vi "FINAL PROJECT PRO .vi"() -> ()   [LabVIEW 2015]
uses:
  <vilib>/LabVIEW Interface for Arduino/Type Defs/Board Type.ctl
  <vilib>/LabVIEW Interface for Arduino/Type Defs/Connection Type.ctl
  <vilib>/LabVIEW Interface for Arduino/Type Defs/Pin Mode.ctl
  <vilib>/Instr/_visa.llb/VISA Configure Serial Port (Instr).vi
  <vilib>/LabVIEW Interface for Arduino/LabVIEW Interface for Arduino.lvlib
panel:
  out "DISPLAY MESSAGE":string
  out "TRANSACTION PROCESSING":string
  out "ARDUINO GREEN":bool
  in  "stop":bool
  out "EMAIL CTRL SIGNAL":bool
  in  "Attachment - Optional":path
  in  "CC (Carbon Copy Recipients - Optional)":string
  out "VIOLATION":bool
  out "TRUCK FIN":bool
  out "CAR FIN":bool
  out "BIKE FIN":bool
  out "TRUCK RFID":bool
  out "CAR RFID":bool
  out "BIKE RFID":bool
  out "identification number":string
  in  "stop 3":bool
  out "Numeric 2":dbl
  out "Waveform Chart 2":dbl(graph)
  out "Numeric 3":dbl
  out "Waveform Chart 3":dbl(graph)
  out "Numeric 4":dbl
  out "Waveform Chart 4":dbl(graph)
  out "Numeric 5":dbl
  out "Waveform Chart 5":dbl(graph)
  out "PIEZOELECTRIC 1":bool
  out "PIEZOELECTRIC 2":bool
  out "PIEZOELECTRIC 3":bool
  out "PIEZOELECTRIC 4":bool
  out "TRUCK":bool
  out "CAR":bool
  out "BIKE":bool
  in  "stop 2":bool
  in  "stop 5":bool
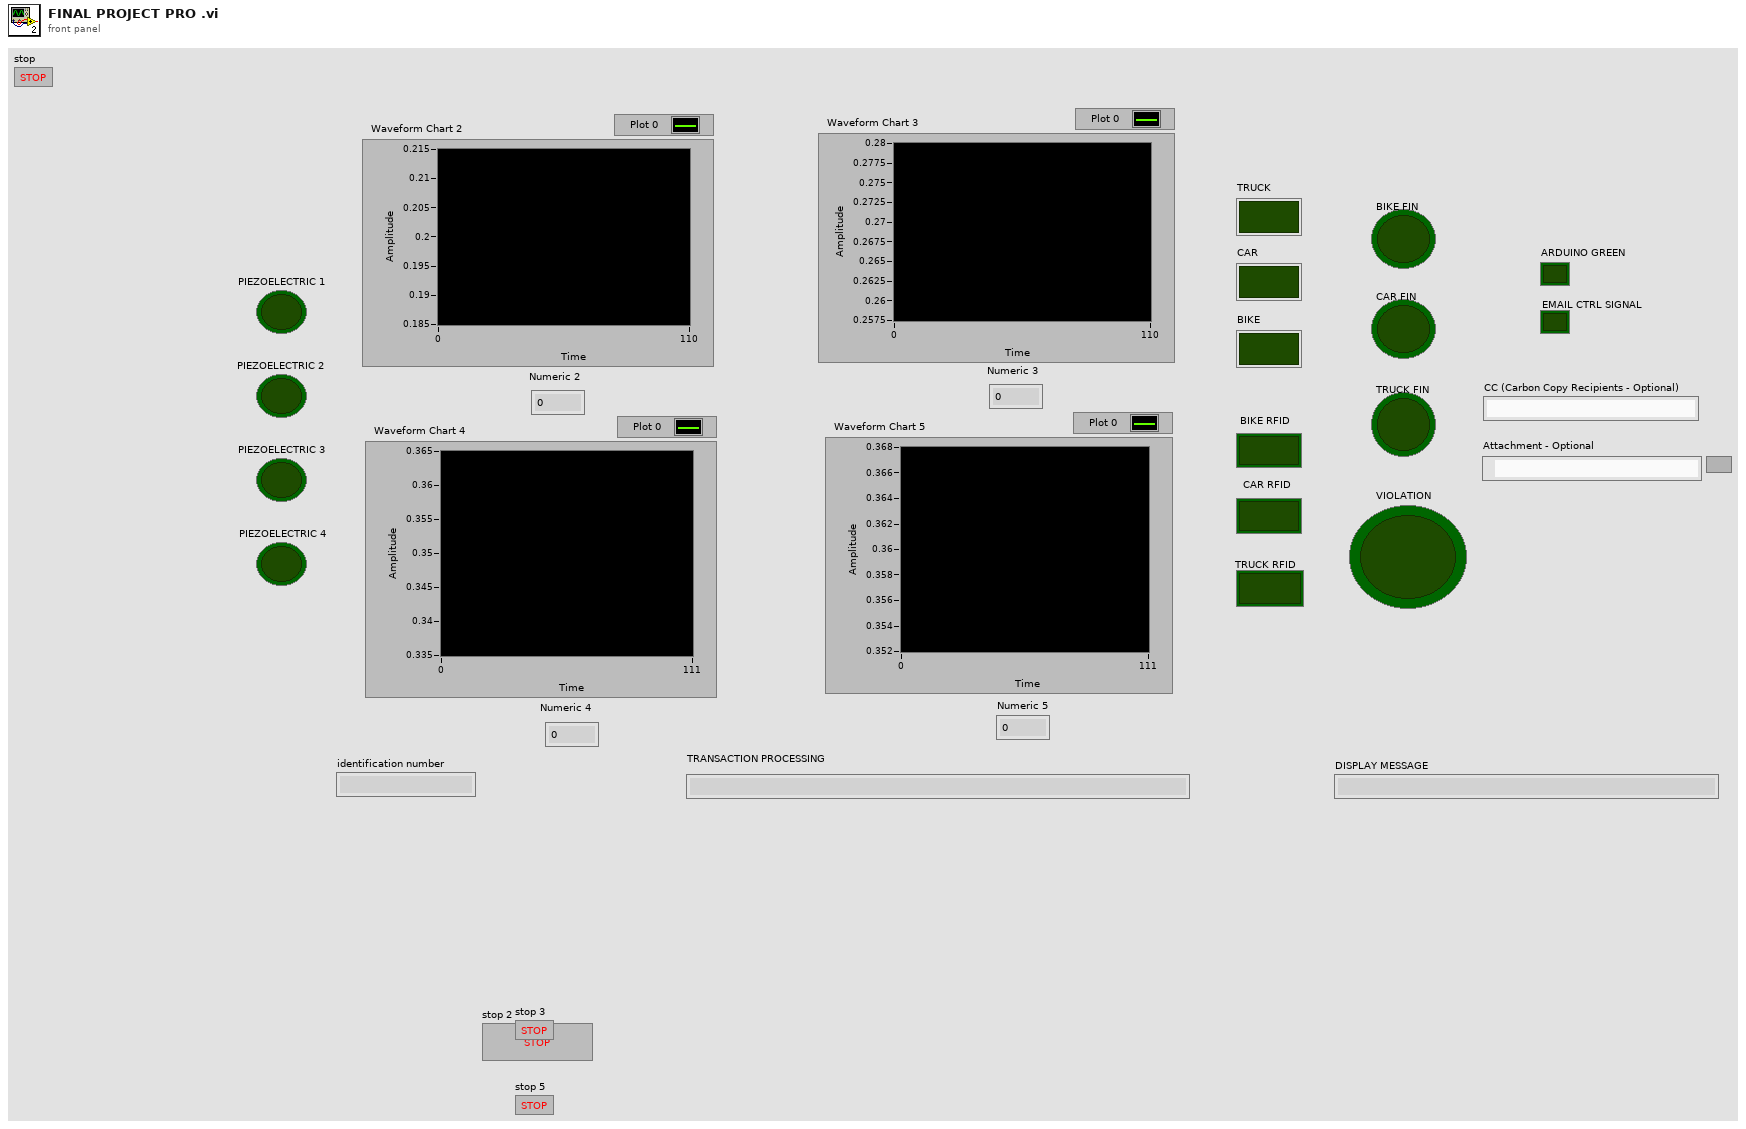
[diagram p1: front panel]
types:
  T1 = typedef "LabVIEW Interface for Arduino.lvlib/Pin Mode.ctl" = enum8{"Input", "Output"}
  T2 = typedef "LabVIEW Interface for Arduino.lvlib/Connection Type.ctl" = enum8{"USB / Serial", "XBEE", "BlueSmirf (Bluetooth)"}
  T3 = typedef "LabVIEW Interface for Arduino.lvlib/Board Type.ctl" = enum16{"Uno", "Dimuelanove w/Atmega 328", "Mega 2560"}
  T4 = typedef "LabVIEW Interface for Arduino.lvlib/Arduino Resource.ctl" = cluster{"VISA resource":refnum<visa-resource-name>, "Board Type":T3, "Connection Type":enum8{"USB / Serial"}, "Bytes Per Packet (15)":u8}
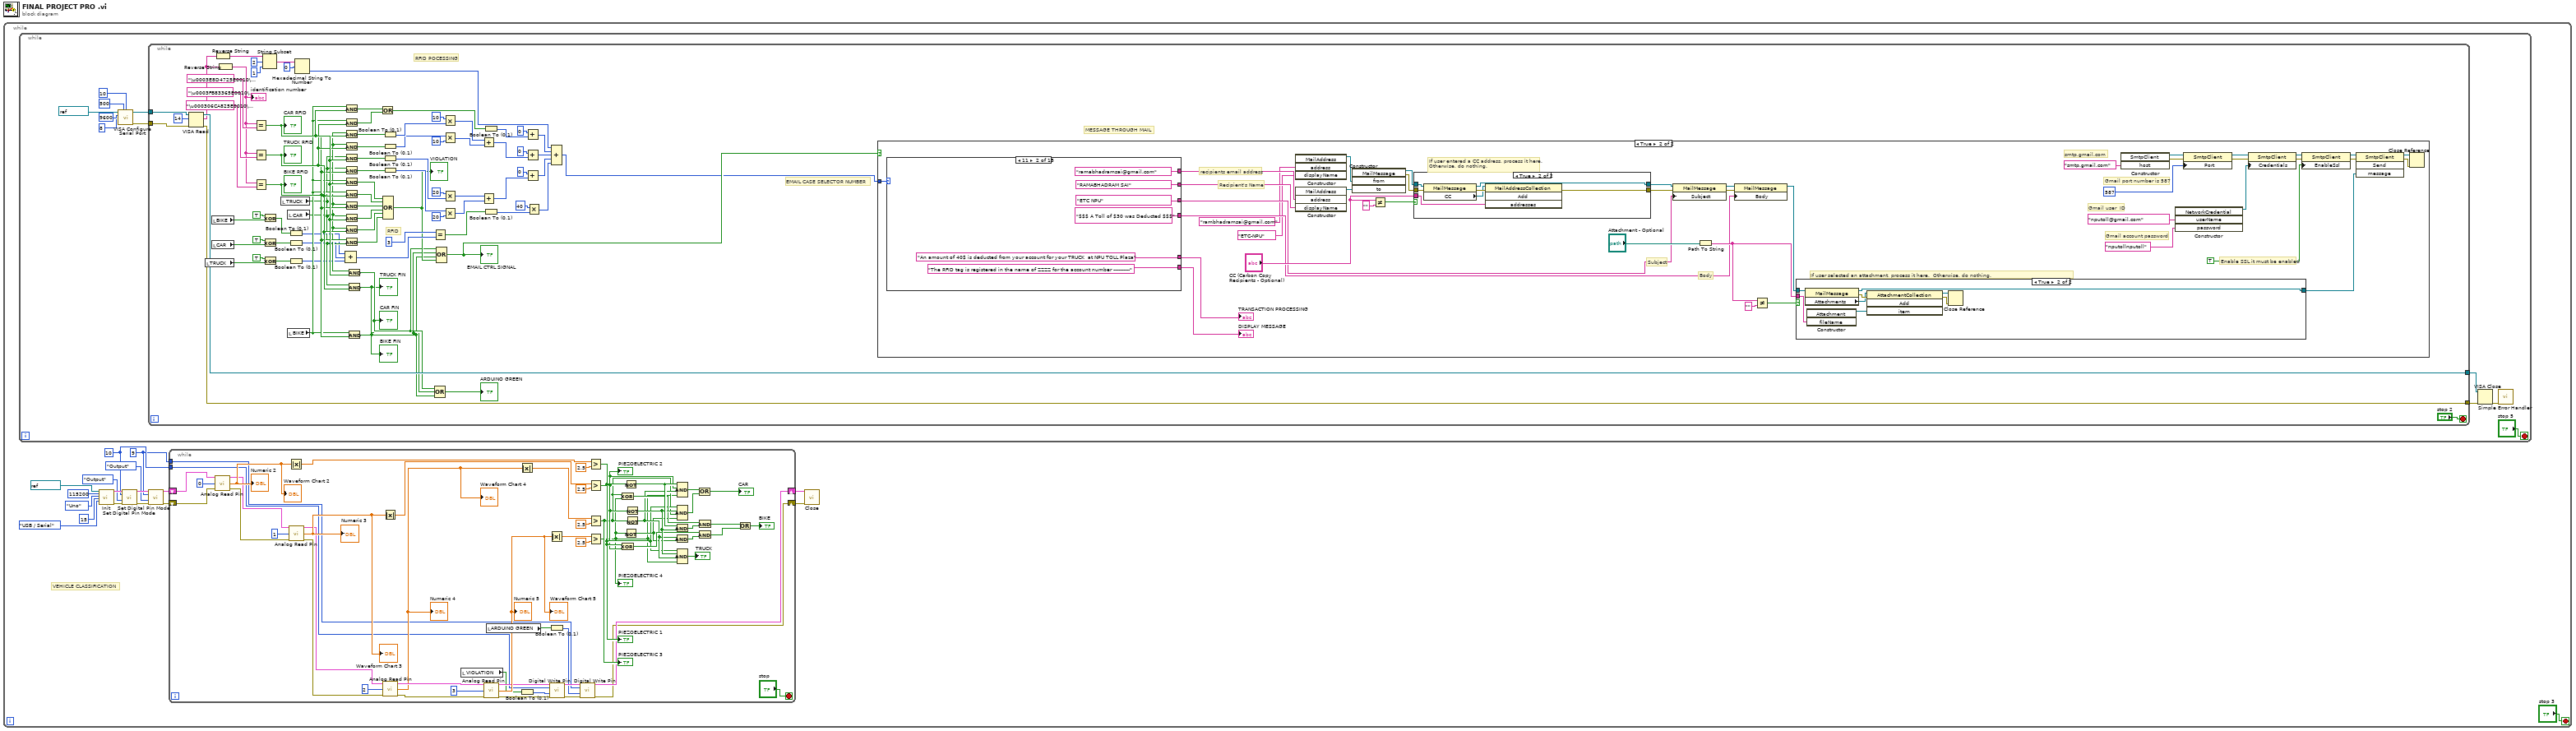
[diagram p0: block diagram]
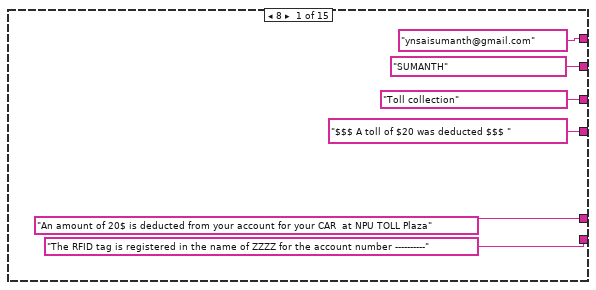
[diagram p3: hidden frame]
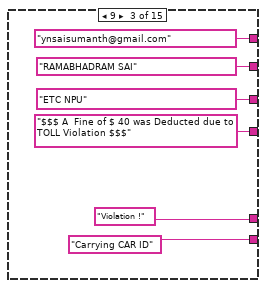
[diagram p4: hidden frame]
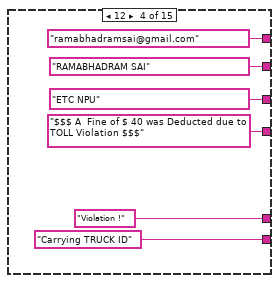
[diagram p5: hidden frame]
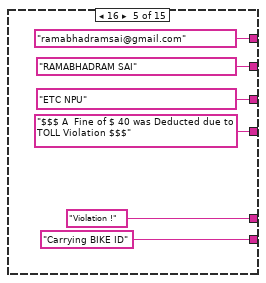
[diagram p6: hidden frame]
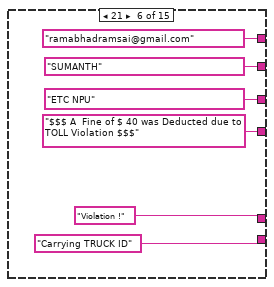
[diagram p7: hidden frame]
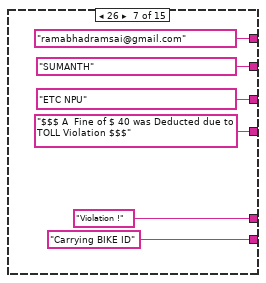
[diagram p8: hidden frame]
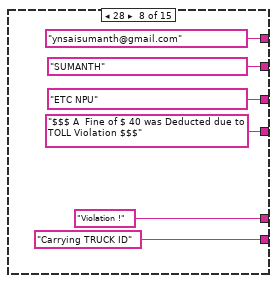
[diagram p9: hidden frame]
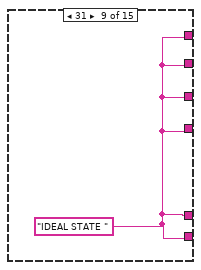
[diagram p10: hidden frame]
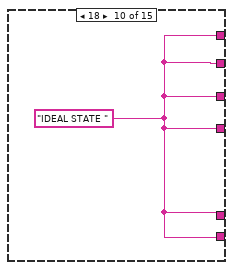
[diagram p11: hidden frame]
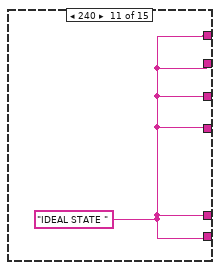
[diagram p12: hidden frame]
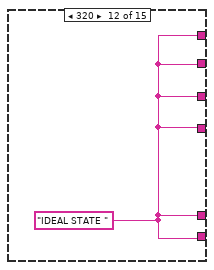
[diagram p13: hidden frame]
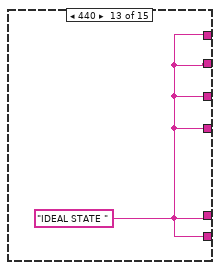
[diagram p14: hidden frame]
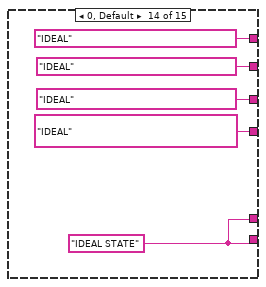
[diagram p15: hidden frame]
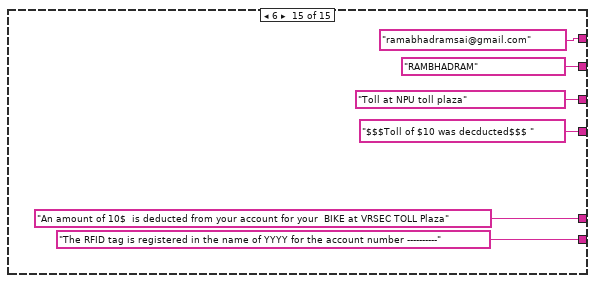
[diagram p16: hidden frame]
diagram:
  n1 = while {
    stop <- "stop 3" stop-if-true
    w2 = u8 10 ("Digital I/O Pin")
    w1 = u8 9 ("Digital I/O Pin")
    # "VEHICLE CLASSIFICATION"
    n2 = while {
      stop <- "stop 5" stop-if-true
      n3 = call-poly "VISA Configure Serial Port"("VISA resource name"=refnum<visa-resource-name> "COM3", "timeout (10sec)"=u32 500, "termination char\n(0xA = '\\n' = LF)"=u8 10 ("termination char\n(0xA = '\\n' = LF)"), "baud rate (9600)"=u32 9600, "data bits (8)"=u16 8) -> ("VISA resource name out"=w81:refnum<visa-resource-name>, "error out"=w80:errorcluster)  [unwired: 9 in]
      n4 = while {
        tunnel: w81 -> [w167]
        tunnel: w80 -> [w166]
        tunnel: [w165] -> w79
        tunnel: [w158] -> w75
        stop <- "stop 2" stop-if-true
        # "MESSAGE THROUGH MAIL"
        # "RFID POCESSING"
        # "RFID"
        # "EMAIL CASE SELECTOR NUMBER"
        n5 = VISA Read(VISA resource name=w167, byte count=u32 14, error in (no error)=w166) -> (VISA resource name out=w158:refnum<visa-resource-name>, read buffer=w146:string, error out=w165:errorcluster)  [unwired: 1 out]
        n6 = local read "TRUCK"() -> (w100:bool)
        n7 = local read "BIKE"() -> (w107:bool)
        n8 = local read "CAR"() -> (w102:bool)
        n9 = Reverse String(1:w146) -> (0:w157:string)
        n10 = Reverse String(1:w146) -> (0:w153:string)
        "identification number" <- w153
        n11 = Equal?(x=w153, y="\u0003E8D4725E0010\u0002") -> (x = y?=w117:bool)
        "CAR RFID" <- w117
        n12 = Equal?(x=w153, y="\u0003FB83365E0010\u0002") -> (x = y?=w116:bool)
        "TRUCK RFID" <- w116
        n13 = Equal?(x=w153, y="\u000306CA825E0010\u0002") -> (x = y?=w115:bool)
        "BIKE RFID" <- w115
        n14 = String Subset(string=w157, offset (0)=2, length (rest)=1 ("length (rest)")) -> (substring=w159:string)
        n15 = Exclusive Or(1:w107, 2:TRUE ("x")) -> (0:w105:bool)
        n16 = Exclusive Or(1:w102, 2:TRUE ("x")) -> (0:w99:bool)
        n17 = Exclusive Or(1:w100, 2:TRUE ("x")) -> (0:w98:bool)
        n18 = local read "TRUCK"() -> (w112:bool)
        n19 = local read "CAR"() -> (w113:bool)
        n20 = local read "BIKE"() -> (w114:bool)
        n21 = Boolean To (0,1)(Boolean=w105) -> (0, 1=w104:i16)
        n22 = Boolean To (0,1)(Boolean=w99) -> (0, 1=w96:i16)
        n23 = Boolean To (0,1)(Boolean=w98) -> (0, 1=w97:i16)
        n24 = Hexadecimal String To Number(string=w159, offset=0) -> (number=w111:u32)  [unwired: 1 in, 1 out]
        n25 = And(x=w114, y=w117) -> (x .and. y?=w142:bool)
        n26 = And(x=w114, y=w116) -> (x .and. y?=w141:bool)
        n27 = And(x=w113, y=w115) -> (x .and. y?=w137:bool)
        n28 = And(x=w113, y=w116) -> (x .and. y?=w134:bool)
        n29 = And(x=w112, y=w117) -> (x .and. y?=w118:bool)
        n30 = And(x=w112, y=w115) -> (x .and. y?=w119:bool)
        n31 = And(x=w114, y=w117) -> (x .and. y?=w152:bool)
        n32 = And(x=w114, y=w116) -> (x .and. y?=w151:bool)
        n33 = And(x=w113, y=w115) -> (x .and. y?=w150:bool)
        n34 = And(x=w112, y=w117) -> (x .and. y?=w149:bool)
        n35 = And(x=w113, y=w116) -> (x .and. y?=w148:bool)
        n36 = And(x=w115, y=w112) -> (x .and. y?=w147:bool)
        n37 = Compound Arithmetic op=ADD(w104, w96, w97) -> (w108:i16)
        n38 = And(x=w113, y=w117) -> (x .and. y?=w90:bool)
        "CAR FIN" <- w90
        n39 = And(x=w112, y=w116) -> (x .and. y?=w89:bool)
        "TRUCK FIN" <- w89
        n40 = And(x=w114, y=w115) -> (x .and. y?=w88:bool)
        "BIKE FIN" <- w88
        n41 = Or(x=w142, y=w141) -> (x .or. y?=w140:bool)
        n42 = Compound Arithmetic op=OR(w152, w151, w150, w149, w148, w147) -> (w92:bool)
        "VIOLATION" <- w92
        n43 = Boolean To (0,1)(Boolean=w137) -> (0, 1=w136:i16)
        n44 = Boolean To (0,1)(Boolean=w134) -> (0, 1=w133:i16)
        n45 = Boolean To (0,1)(Boolean=w118) -> (0, 1=w122:i16)
        n46 = Boolean To (0,1)(Boolean=w119) -> (0, 1=w124:i16)
        n47 = Equal?(x=3, y=w108) -> (x = y?=w109:bool)
        n48 = Compound Arithmetic op=OR(w90, w89, w88) -> (→"ARDUINO GREEN":bool)
        n49 = Compound Arithmetic op=OR(w90, w89, w88, w92) -> (w91:bool)
        "EMAIL CTRL SIGNAL" <- w91
        n50 = Multiply(x=i16 10, y=w136) -> (x*y=w131:i16)
        n51 = Multiply(x=w133, y=i16 10) -> (x*y=w130:i16)
        n52 = Multiply(x=i16 20, y=w122) -> (x*y=w126:i16)
        n53 = Multiply(x=w124, y=i16 20) -> (x*y=w127:i16)
        n54 = Add(x=w131, y=w130) -> (x+y=w129:i16)
        n55 = Add(x=w126, y=w127) -> (x+y=w128:i16)
        n56 = Boolean To (0,1)(Boolean=w140) -> (0, 1=w145:i16)
        n57 = Boolean To (0,1)(Boolean=w109) -> (0, 1=w95:i16)
        n58 = Add(x=i16 0, y=w145) -> (x+y=w143:i16)
        n59 = Add(x=i16 0, y=w129) -> (x+y=w138:i16)
        n60 = Add(x=i16 0, y=w128) -> (x+y=w120:i16)
        n61 = Multiply(x=40, y=w95) -> (x*y=w93:i32)
        n62 = Compound Arithmetic op=ADD(w111, w143, w138, w120, w93) -> (w86:u32)
        n63 = case shown="True" w91 {
          tunnel: w86 -> [_ w177]
          frame False {
          }
          frame True {
            # "Enable SSL it must be enabled"
            # "Gmail port number is 587"
            # "Gmail account password"
            # "Gmail user  ID"
            # "smtp.gmail.com"
            # "Body"
            # "Subject"
            # "Recipient's Name"
            # "recipients email address"
            # "If user selected an attachment, process it here.  Otherwise, do nothing."
            # "If user entered a CC address, process it here.\nOtherwise, do nothing."
            n64 = case shown="11" w177 {
              tunnel: ["ynsaisumanth@gmail.com" "ramabhadramsai@gmail.com" "ynsaisumanth@gmail.com" "ramabhadramsai@gmail.com" "ramabhadramsai@gmail.com" "ramabhadramsai@gmail.com" "ramabhadramsai@gmail.com" "ynsaisumanth@gmail.com" w258 w259 w260 w261 w262 "IDEAL" "ramabhadramsai@gmail.com"] -> w181
              tunnel: ["SUMANTH" "RAMABHADRAM SAI" "RAMABHADRAM SAI" "RAMABHADRAM SAI" "RAMABHADRAM SAI" "SUMANTH" "SUMANTH" "SUMANTH" w258 w259 w260 w261 w262 "IDEAL" "RAMBHADRAM"] -> w180
              tunnel: ["Toll collection" "ETC NPU" "ETC NPU" "ETC NPU" "ETC NPU" "ETC NPU" "ETC NPU" "ETC NPU" w258 w259 w260 w261 w262 "IDEAL" "Toll at NPU toll plaza"] -> w179
              tunnel: ["$$$ A toll of $20 was deducted $$$ " "$$$ A Toll of $30 was Deducted $$$" "$$$ A  Fine of $ 40 was Deducted due to TOLL Violation $$$" "$$$ A  Fine of $ 40 was Deducted due to TOLL Violation $$$" "$$$ A  Fine of $ 40 was Deducted due to TOLL Violation $$$" "$$$ A  Fine of $ 40 was Deducted due to TOLL Violation $$$" "$$$ A  Fine of $ 40 was Deducted due to TOLL Violation $$$" "$$$ A  Fine of $ 40 was Deducted due to TOLL Violation $$$" w258 w259 w260 w261 w262 "IDEAL" "$$$Toll of $10 was decducted$$$ "] -> w178
              tunnel: ["An amount of 20$ is deducted from your account for your CAR  at NPU TOLL Plaza" ("Amount deducted") "An amount of 40$ is deducted from your account for your TRUCK  at NPU TOLL Plaza" ("Amount deducted") "Violation !" ("Amount deducted") "Violation !" ("Amount deducted") "Violation !" ("Amount deducted") "Violation !" ("Amount deducted") "Violation !" ("Amount deducted") "Violation !" ("Amount deducted") w258 w259 w260 w261 w262 w263 "An amount of 10$  is deducted from your account for your  BIKE at VRSEC TOLL Plaza" ("Amount deducted")] -> w169
              tunnel: ["The RFID tag is registered in the name of ZZZZ for the account number ----------" "The RFID tag is registered in the name of ZZZZ for the account number ----------" "Carrying CAR ID" ("Amount deducted") "Carrying TRUCK ID" ("Amount deducted") "Carrying BIKE ID" ("Amount deducted") "Carrying TRUCK ID" ("Amount deducted") "Carrying BIKE ID" ("Amount deducted") "Carrying TRUCK ID" ("Amount deducted") w258 w259 w260 w261 w262 w263 "The RFID tag is registered in the name of YYYY for the account number ----------"] -> w168
              frame 8 {
              }
              frame 11 {
              }
              frame 9 {
              }
              frame 12 {
              }
              frame 16 {
              }
              frame 21 {
              }
              frame 26 {
              }
              frame 28 {
              }
              frame 31 {
                w258 = "IDEAL STATE "
              }
              frame 18 {
                w259 = "IDEAL STATE "
              }
              frame 240 {
                w260 = "IDEAL STATE "
              }
              frame 320 {
                w261 = "IDEAL STATE "
              }
              frame 440 {
                w262 = "IDEAL STATE "
              }
              frame 0, Default {
                w263 = "IDEAL STATE" ("Amount deducted")
              }
              frame 6 {
              }
            }
            "TRANSACTION PROCESSING" <- w169
            "DISPLAY MESSAGE" <- w168
            n65 = constructor class="MailAddress"("address"="rambhadramsai@gmail.com", "displayName"="ETC-NPU") -> (reference out=w208:refnum<k24>)  [unwired: 3 in, 4 out]
            n66 = constructor class="MailAddress"("address"=w181, "displayName"=w180) -> (reference out=w209:refnum<k24>)  [unwired: 3 in, 4 out]
            n67 = constructor class="MailMessage"("from"=w208, "to"=w209) -> (reference out=w187:refnum<k24>, error out=w186:errorcluster)  [unwired: 3 in, 3 out]
            n68 = Not Equal?(x="CC (Carbon Copy Recipients - Optional)", y="") -> (x != y?=w189:bool)
            n69 = case shown="True" w189 {
              tunnel: "CC (Carbon Copy Recipients - Optional)" -> [_ w280]
              tunnel: w187 -> [w275 w279]
              tunnel: w186 -> [w274 w278]
              tunnel: [w275 w277] -> w185
              tunnel: [w274 w276] -> w184
              frame False {
              }
              frame True {
                n70 = property class="MailMessage"(reference=w279, error in=w278) -> (reference out=w277:refnum<k24>, error out=w282:errorcluster, "CC"=w281:refnum<k24>)
                n71 = invoke class="MailAddressCollection" method="Add"(reference=w281, error in=w282, "addresses"=w280) -> (error out=w276:errorcluster)  [unwired: 1 in, 3 out]
              }
            }
            n72 = property class="MailMessage"(reference=w185, error in=w184, "Subject"=w179) -> (reference out=w206:refnum<k24>, error out=w207:errorcluster)
            n73 = Path To String(path="Attachment - Optional") -> (string=w191:string)
            n74 = property class="MailMessage"(reference=w206, error in=w207, "Body"=w178) -> (reference out=w196:refnum<k24>)  [unwired: 1 out]
            n75 = Not Equal?(x=w191, y="") -> (x != y?=w192:bool)
            n76 = case shown="True" w192 {
              tunnel: w196 -> [w283 w288]
              tunnel: [w283 w287] -> w195
              tunnel: w191 -> [_ w286]
              frame False {
              }
              frame True {
                n77 = property class="MailMessage"(reference=w288) -> (reference out=w287:refnum<k24>, error out=w291:errorcluster, "Attachments"=w289:refnum<k24>)  [unwired: 1 in]
                n78 = constructor class="Attachment"("fileName"=w286) -> (reference out=w290:refnum<k24>)  [unwired: 3 in, 3 out]
                n79 = invoke class="AttachmentCollection" method="Add"(reference=w289, error in=w291, "item"=w290) -> (reference out=w285:refnum<k24>, error out=w284:errorcluster)  [unwired: 1 in, 2 out]
                n80 = Close Reference(reference=w285, error in (no error)=w284) -> ()  [unwired: 1 out]
              }
            }
            n81 = constructor class="SmtpClient"("host"="smtp.gmail.com") -> (reference out=w204:refnum<k24>, error out=w200:errorcluster)  [unwired: 3 in, 2 out]
            n82 = constructor class="NetworkCredential"("userName"="nputoll@gmail.com", "password"="nputollnputoll") -> (reference out=w205:refnum<k24>)  [unwired: 3 in, 4 out]
            n83 = property class="SmtpClient"(reference=w204, error in=w200, "Port"=587) -> (reference out=w203:refnum<k24>, error out=w199:errorcluster)
            n84 = property class="SmtpClient"(reference=w203, error in=w199, "Credentials"=w205) -> (reference out=w202:refnum<k24>, error out=w198:errorcluster)
            n85 = property class="SmtpClient"(reference=w202, error in=w198, "EnableSsl"=TRUE) -> (reference out=w201:refnum<k24>, error out=w197:errorcluster)
            n86 = invoke class="SmtpClient" method="Send"(reference=w201, error in=w197, "message"=w195) -> (reference out=w183:refnum<k24>, error out=w182:errorcluster)  [unwired: 1 in, 2 out]
            n87 = Close Reference(reference=w183, error in (no error)=w182) -> ()  [unwired: 1 out]
          }
        }
      }
      n88 = VISA Close(VISA resource name=w75, error in (no error)=w79) -> (error out=w78:errorcluster)
      n89 = call <vilib>:"Simple Error Handler.vi"("error in (no error)"=w78) -> ()  [unwired: 4 in, 5 out]
    }
    n90 = call <vilib>:"Init.vi"("VISA resource"=refnum<visa-resource-name> "COM4", "Baud Rate (115200)"=u32 115200, "Board Type (Uno)"=Board_Type."Uno", "Bytes Per Packet (15)"=u32 15, "Connection Type (USB/Serial)"=Connection_Type."USB / Serial") -> ("Arduino Resource"=w10:T4, "error out"=w7:errorcluster)  [unwired: 13 in]
    n91 = call <vilib>:"Set Digital Pin Mode.vi"("Arduino Resource"=w10, "Digital I/O Pin"=w2, "Pin Mode (Input)"=Pin_Mode."Output", "error in"=w7) -> ("Arduino Resource"=w9:T4, "error out"=w6:errorcluster)  [unwired: 10 in]
    n92 = call <vilib>:"Set Digital Pin Mode.vi"("Arduino Resource"=w9, "Digital I/O Pin"=w1, "Pin Mode (Input)"=Pin_Mode."Output", "error in"=w6) -> ("Arduino Resource"=w8:T4, "error out"=w5:errorcluster)  [unwired: 10 in]
    n93 = while {
      shift-right: [w28] -> w12
      shift-left: w8 -> [w74]
      shift-right: [w27] -> w11
      shift-left: w5 -> [w73]
      tunnel: w2 -> [w24]
      tunnel: w1 -> [w23]
      stop <- "stop" stop-if-true
      n94 = call <vilib>:"Analog Read Pin.vi"("Arduino Resource"=w74, "Analog Input Pin (0)"=u8 0, "error in"=w73) -> ("Arduino Resource"=w42:T4, "Voltage"=w45:dbl, "error out"=w41:errorcluster)  [unwired: 10 in]
      "Numeric 2" <- w45
      "Waveform Chart 2" <- w45
      n95 = Absolute Value(x=w45) -> (abs(x)=w49:dbl)
      n96 = call <vilib>:"Analog Read Pin.vi"("Arduino Resource"=w42, "Analog Input Pin (0)"=u8 1, "error in"=w41) -> ("Arduino Resource"=w40:T4, "Voltage"=w44:dbl, "error out"=w39:errorcluster)  [unwired: 10 in]
      "Numeric 3" <- w44
      "Waveform Chart 3" <- w44
      n97 = Absolute Value(x=w44) -> (abs(x)=w48:dbl)
      n98 = call <vilib>:"Analog Read Pin.vi"("Arduino Resource"=w40, "Analog Input Pin (0)"=u8 2, "error in"=w39) -> ("Arduino Resource"=w38:T4, "Voltage"=w31:dbl, "error out"=w37:errorcluster)  [unwired: 10 in]
      "Numeric 4" <- w31
      "Waveform Chart 4" <- w31
      n99 = local read "VIOLATION"() -> (w22:bool)
      n100 = call <vilib>:"Analog Read Pin.vi"("Arduino Resource"=w38, "Analog Input Pin (0)"=u8 3, "error in"=w37) -> ("Arduino Resource"=w30:T4, "Voltage"=w43:dbl, "error out"=w25:errorcluster)  [unwired: 10 in]
      "Numeric 5" <- w43
      "Waveform Chart 5" <- w43
      n101 = local read "ARDUINO GREEN"() -> (w19:bool)
      n102 = Absolute Value(x=w31) -> (abs(x)=w47:dbl)
      n103 = Boolean To (0,1)(Boolean=w22) -> (0, 1=w21:i16)
      n104 = Absolute Value(x=w43) -> (abs(x)=w46:dbl)
      n105 = Boolean To (0,1)(Boolean=w19) -> (0, 1=w20:i16)
      n106 = call <vilib>:"Digital Write Pin.vi"("Arduino Resource"=w30, "Digital I/O Pin (0)"=w24, "Value (0)"=w21, "error in"=w25) -> ("Arduino Resource"=w29:T4, "error out"=w26:errorcluster)  [unwired: 10 in]
      n107 = call <vilib>:"Digital Write Pin.vi"("Arduino Resource"=w29, "Digital I/O Pin (0)"=w23, "Value (0)"=w20, "error in"=w26) -> ("Arduino Resource"=w28:T4, "error out"=w27:errorcluster)  [unwired: 10 in]
      n108 = Greater?(x=w49, y=2.5) -> (0:w60:bool)
      "PIEZOELECTRIC 1" <- w60
      n109 = Greater?(x=w48, y=2.5) -> (0:w59:bool)
      "PIEZOELECTRIC 2" <- w59
      n110 = Greater?(x=w47, y=2.5) -> (0:w58:bool)
      "PIEZOELECTRIC 3" <- w58
      n111 = Greater?(x=w46, y=2.5) -> (0:w57:bool)
      "PIEZOELECTRIC 4" <- w57
      n112 = Exclusive Or(1:w57, 2:w58) -> (0:w68:bool)
      n113 = Exclusive Or(1:w59, 2:w60) -> (0:w65:bool)
      n114 = Not(x=w60) -> (.not. x?=w70:bool)
      n115 = Not(x=w57) -> (.not. x?=w63:bool)
      n116 = Not(x=w59) -> (.not. x?=w69:bool)
      n117 = Not(x=w58) -> (.not. x?=w64:bool)
      n118 = And(x=w70, y=w69) -> (x .and. y?=w67:bool)
      n119 = And(x=w64, y=w63) -> (x .and. y?=w66:bool)
      n120 = Compound Arithmetic op=AND(w70, w59, w64, w57) -> (w72:bool)
      n121 = Compound Arithmetic op=AND(w60, w69, w58, w63) -> (w71:bool)
      n122 = Compound Arithmetic op=AND(w60, w69, w64, w57) -> (→"TRUCK":bool)
      n123 = Or(x=w72, y=w71) -> (x .or. y?=→"CAR":bool)
      n124 = And(x=w68, y=w67) -> (x .and. y?=w62:bool)
      n125 = And(x=w65, y=w66) -> (x .and. y?=w61:bool)
      n126 = Or(x=w62, y=w61) -> (x .or. y?=→"BIKE":bool)
    }
    n127 = call <vilib>:"Close.vi"("Arduino Resource"=w12, "error in"=w11) -> ()  [unwired: 13 in, 1 out]
  }
